vi "GetCamera.vi"(3 "error out 2":errorcluster) -> (12 "CCD Chip horizontal end":i32, 14 "CCD Chip Vertical end":i32, 16 "array":i32[][](array[numeric]), 17 "error out":errorcluster, 18 "low":i32, 19 "high":i32, 27 "kinetic":sgl format="%.2f")   [LabVIEW 2013]
uses:
  lib/atmcd32d.llb/ReadMode_mode typedef.ctl
  lib/atmcd32d.llb/TriggerMode_mode typedef.ctl
  lib/atmcd32d.llb/Shutter_type typedef.ctl
  lib/atmcd32d.llb/Shutter_mode typedef.ctl
  lib/atmcd32d.llb/HSSpeed_type typedef.ctl
  lib/atmcd32d.llb/EMGainMode_mode typedef.ctl
  lib/atmcd32d.llb/Spool_method typedef.ctl
  lib/atmcd32d.llb/Error Code Enum typedef.ctl
  lib/atmcd32d.llb/AcquisitionMode_mode typedef.ctl
  Variables/GlobalSetGetConfigureCamera.vi
  Variables/ccdChipPixels.vi
  Variables/MesaurementModus.vi
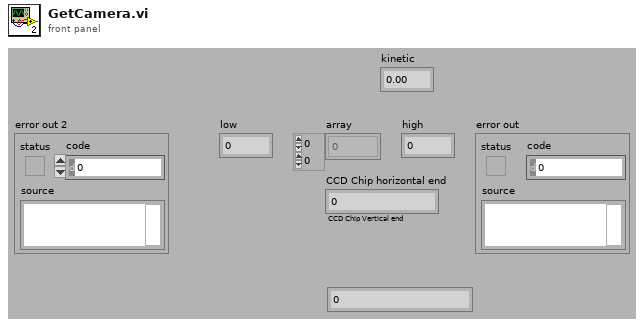
[diagram p1: front panel]
types:
  T1 = typedef "Spool_method typedef.ctl" = enum16{"32-bit", "Depends", "16-bit", "Multiple Directory", "Spool to RAM disk", "16-bit FITS", "SIF", "16-buit TIFF", "Multiple Directory Compressed"}
  T2 = typedef "EMGainMode_mode typedef.ctl" = enum16{"8-bit", "12-bit", "Linear", "Real"}
  T3 = typedef "HSSpeed_type typedef.ctl" = enum16{"EM Amp", "Conventional Amp"}
  T4 = typedef "Shutter_mode typedef.ctl" = enum16{"Auto", "Open", "Close"}
  T5 = typedef "Shutter_type typedef.ctl" = enum16{"TTL Low", "TTL High"}
  T6 = typedef "TriggerMode_mode typedef.ctl" = enum16{"Internal", "External", "N/A (2)", "N/A (3)", "N/A (4)", "N/A (5)", "External Start"}
  T7 = typedef "ReadMode_mode typedef.ctl" = enum16{"Full Vertical Binning", "Multi-Track", "Random-Track", "Single-Track", "Image"}
  T8 = typedef "AcquisitionMode_mode typedef.ctl" = enum16{"Reserved (0)", "Single Scan", "Accumulate", "Kinetics", "Fast Kinetics", "Run Till Abort", "Reserved (6)", "Reserved (7)", "Reserved (8)", "Time Delayed Integration"}
  T9 = typedef "Error Code Enum typedef.ctl" = enum32{"N/A (0)", "DRV_ERROR_CODES", "DRV_SUCCESS", "DRV_VXDNOTINSTALLED", "DRV_ERROR_SCAN", "DRV_ERROR_CHECK_SUM", "DRV_ERROR_FILELOAD", "DRV_UNKNOWN_FUNC", "DRV_ERROR_VXD_INIT", "DRV_ERROR_ADDRESS", "DRV_ERROR_PAGELOCK", "DRV_ERROR_PAGEUNLOCK", "DRV_ERROR_BOARDTEST", "DRV_ERROR_ACK", "DRV_ERROR_UP_FIFO", "DRV_ERROR_PATTERN", "N/A (16)", "DRV_ACQUISITION_ERRORS", "DRV_ACQ_BUFFER", "DRV_ACQ_DOWNFIFO_FULL", "DRV_PROC_UNKONWN_INSTRUCTION", "DRV_ILLEGAL_OP_CODE", "DRV_KINETIC_TIME_NOT_MET", "DRV_ACCUM_TIME_NOT_MET", "DRV_NO_NEW_DATA", "N/A (25)", "DRV_SPOOLERROR", "N/A (27)", "N/A (28)", "N/A (29)", "N/A (30)", "N/A (31)", "N/A (32)", "DRV_TEMPERATURE_CODES", "DRV_TEMPERATURE_OFF", "DRV_TEMPERATURE_NOT_STABILIZED", "DRV_TEMPERATURE_STABILIZED", "DRV_TEMPERATURE_NOT_REACHED", "DRV_TEMPERATURE_OUT_RANGE", "DRV_TEMPERATURE_NOT_SUPPORTED", "DRV_TEMPERATURE_DRIFT", "N/A (41)", "N/A (42)", "N/A (43)", "N/A (44)", "N/A (45)", "N/A (46)", "N/A (47)", "N/A (48)", "DRV_GENERAL_ERRORS", "DRV_INVALID_AUX", "DRV_COF_NOTLOADED", "DRV_FPGAPROG", "DRV_FLEXERROR", "DRV_GPIBERROR", "N/A (55)", "N/A (56)", "N/A (57)", "N/A (58)", "N/A (59)", "N/A (60)", "N/A (61)", "N/A (62)", "N/A (63)", "DRV_DATATYPE", "DRV_DRIVER_ERRORS", "DRV_P1INVALID", "DRV_P2INVALID", "DRV_P3INVALID", "DRV_P4INVALID", "DRV_INIERROR", "DRV_COFERROR", "DRV_ACQUIRING", "DRV_IDLE", "DRV_TEMPCYCLE", "DRV_NOT_INITIALIZED", "DRV_P5INVALID", "DRV_P6INVALID", "DRV_INVALID_MODE", "DRV_INVALID_FILTER", "DRV_I2CERRORS", "DRV_I2CDEVNOTFOUND", "DRV_I2CTIMEOUT", "DRV_P7INVALID", "N/A (84)", "N/A (85)", "N/A (86)", "N/A (87)", "N/A (88)", "N/A (89)", "DRV_IOCERROR", "DRV_VRMVERSIONERROR"}
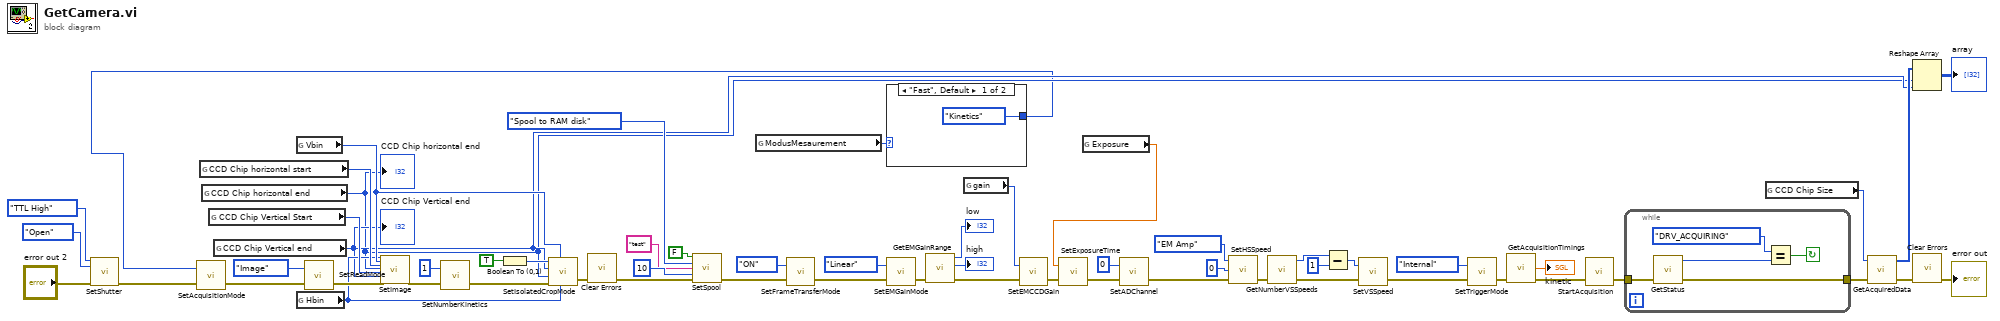
[diagram p0: block diagram]
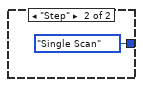
[diagram p2: hidden frame]
diagram:
  n1 = call "SetShutter.vi"("type"=Shutter_type_typedef."TTL High", "mode"=Shutter_mode_typedef."Open", "error in (no error)"="error out 2") -> ("error out"=w54:errorcluster)  [unwired: 11 in, 1 out]
  n2 = global read "ccdChipPixels.vi" "CCD Chip horizontal start"() -> (w29:i32)
  n3 = global read "ccdChipPixels.vi" "CCD Chip horizontal end"() -> (w13:i32)
  "CCD Chip horizontal end" <- w13
  n4 = global read "ccdChipPixels.vi" "CCD Chip Vertical Start"() -> (w30:i32)
  n5 = global read "ccdChipPixels.vi" "CCD Chip Vertical end"() -> (w14:i32)
  "CCD Chip Vertical end" <- w14
  n6 = global read "GlobalSetGetConfigureCamera.vi" "Vbin"() -> (w16:i32)
  n7 = global read "GlobalSetGetConfigureCamera.vi" "Hbin"() -> (w15:i32)
  n8 = Boolean To (0,1)(Boolean=TRUE) -> (0, 1=w20:i16)
  n9 = global read "MesaurementModus.vi" "ModusMesaurement"() -> (w3:enum32{"Fast", "Step"})
  n10 = case shown="\"Fast\", Default" w3 {
    tunnel: [AcquisitionMode_mode_typedef."Kinetics" ("mode") AcquisitionMode_mode_typedef."Single Scan" ("mode")] -> w2
    frame "Fast", Default {
    }
    frame "Step" {
    }
  }
  n11 = call "SetAcquisitionMode.vi"("error in (no error)"=w54, "mode"=w2) -> ("error out"=w31:errorcluster)  [unwired: 1 out]
  n12 = call "SetReadMode.vi"("error in (no error)"=w31, "mode"=ReadMode_mode_typedef."Image") -> ("error out"=w32:errorcluster)  [unwired: 1 out]
  n13 = call "SetImage.vi"("hbin"=w15, "vbin"=w16, "hstart"=w29, "hend"=w13, "vstart"=w30, "vend"=w14, "error in (no error)"=w32) -> ("error out"=w58:errorcluster)  [unwired: 19 in, 1 out]
  n14 = call "SetNumberKinetics.vi"("error in (no error)"=w58, "number"=1) -> ("error out"=w19:errorcluster)  [unwired: 1 out]
  n15 = call "SetIsolatedCropMode.vi"("hbin"=w15, "vbin"=w16, "error in (no error)"=w19, "cropWidth"=w13, "cropHeight"=w14, "active"=w20) -> ("error out"=w12:errorcluster)  [unwired: 1 out]
  n16 = call <vilib>:"Clear Errors.vi"("error in (no error)"=w12) -> ("error out"=w11:errorcluster)  [unwired: 6 in]
  n17 = call "SetSpool.vi"("active"=FALSE, "method"=Spool_method_typedef."Spool to RAM disk", "name"="test", "framebuffersize (10)"=10, "error in (no error)"=w11) -> ("error out"=w18:errorcluster)  [unwired: 9 in, 1 out]
  n18 = call "SetFrameTransferMode.vi"("error in (no error)"=w18, "mode"=enum16{"OFF", "ON"}."ON") -> ("error out"=w17:errorcluster)  [unwired: 1 out]
  n19 = call "SetEMGainMode.vi"("error in (no error)"=w17, "mode"=EMGainMode_mode_typedef."Linear") -> ("error out"=w50:errorcluster)  [unwired: 1 out]
  n20 = call "GetEMGainRange.vi"("error in (no error)"=w50) -> ("error out"=w51:errorcluster, "high"=→"high":i32, "low"=→"low":i32)  [unwired: 3 in, 1 out]
  n21 = global read "GlobalSetGetConfigureCamera.vi" "gain"() -> (w28:i32)
  n22 = call "SetEMCCDGain.vi"("error in (no error)"=w51, "gain"=w28) -> ("error out"=w49:errorcluster)  [unwired: 1 out]
  n23 = global read "GlobalSetGetConfigureCamera.vi" "Exposure"() -> (w1:sgl)
  n24 = call "SetExposureTime.vi"("error in (no error)"=w49, "time"=w1) -> ("error out"=w33:errorcluster)  [unwired: 1 out]
  n25 = call "SetADChannel.vi"("error in (no error)"=w33, "channel"=0) -> ("error out"=w34:errorcluster)  [unwired: 1 out]
  n26 = call "SetHSSpeed.vi"("error in (no error)"=w34, "index"=0, "type"=HSSpeed_type_typedef."EM Amp") -> ("error out"=w38:errorcluster)  [unwired: 1 in, 1 out]
  n27 = call "GetNumberVSSpeeds.vi"("error in (no error)"=w38) -> ("error out"=w40:errorcluster, "number"=w37:i32)  [unwired: 2 in, 1 out]
  n28 = Subtract(x=w37, y=1) -> (x-y=w35:i32)
  n29 = call "SetVSSpeed.vi"("error in (no error)"=w40, "index"=w35) -> ("error out"=w39:errorcluster)  [unwired: 1 out]
  n30 = call "SetTriggerMode.vi"("error in (no error)"=w39, "mode"=TriggerMode_mode_typedef."Internal") -> ("error out"=w7:errorcluster)  [unwired: 1 out]
  n31 = call "GetAcquisitionTimings.vi"("error in (no error)"=w7) -> ("kinetic"=→"kinetic":sgl, "error out"=w6:errorcluster)  [unwired: 10 in, 3 out]
  n32 = call "StartAcquisition.vi"("error in (no error)"=w6) -> ("error out"=w10:errorcluster)  [unwired: 1 in, 1 out]
  n33 = while {
    tunnel: w10 -> [w66]
    tunnel: [w65] -> w9
    stop <- w62 continue-if-true
    n34 = call "GetStatus.vi"("error in (no error)"=w66) -> ("error out"=w65:errorcluster, "status"=w63:T9)  [unwired: 2 in, 1 out]
    n35 = Equal?(x=Error_Code_Enum_typedef."DRV_ACQUIRING" ("status"), y=w63) -> (x = y?=w62:bool)
  }
  n36 = global read "ccdChipPixels.vi" "CCD Chip Size"() -> (w4:i32)
  n37 = call "GetAcquiredData.vi"("error in (no error)"=w9, "size"=w4) -> ("error out"=w8:errorcluster, "array"=w27:i32[])  [unwired: 1 in, 1 out]
  n38 = Reshape Array(w27, w13, w14) -> (→"array":i32[][])
  n39 = call <vilib>:"Clear Errors.vi"("error in (no error)"=w8) -> ("error out"=→"error out":errorcluster)  [unwired: 6 in]
